vi "Refresh GMaps.vi"(0 "GMaps API in":refnum<class "GMaps API.lvclass">, 1 "Updating String":string, 2 "Automation Refnum in":refnum<k7>, 5 "error in (no error)":errorcluster, 6 "Google Maps API Key":string) -> (14 "GMaps API out":refnum<class "GMaps API.lvclass">, 15 "Updated String":string, 16 "Automation Refnum out":refnum<k7>, 19 "error out":errorcluster)   [LabVIEW 2016, in "GMaps API.lvclass"]
doc: "Refreshes the map when there is a new update of configuration options."
uses:
  GMaps API.lvclass
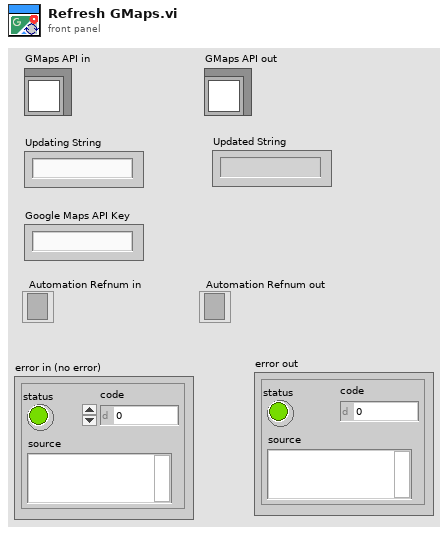
[diagram p1: front panel]
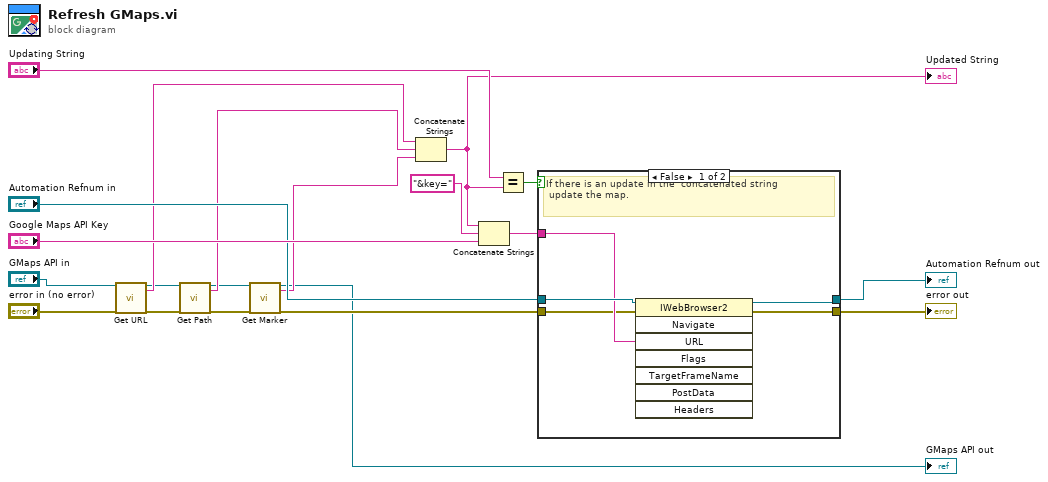
[diagram p0: block diagram]
diagram:
  n1 = call "Get URL.vi"("GMaps API in"="GMaps API in", "error in (no error)"="error in (no error)") -> ("GMaps API out"=w7:refnum<class "GMaps API.lvclass">, "Concateneted URL"=w12:string, "error out"=w5:errorcluster)  [unwired: 15 in]
  n2 = call "Get Path.vi"("GMaps API in"=w7, "error in (no error)"=w5) -> ("GMaps API out"=w6:refnum<class "GMaps API.lvclass">, "Concatenated Path"=w10:string, "error out"=w4:errorcluster)  [unwired: 15 in]
  n3 = call "Get Marker.vi"("GMaps API in"=w6, "error in (no error)"=w4) -> ("GMaps API out"=→"GMaps API out":refnum<class "GMaps API.lvclass">, "Concateneted Marker"=w11:string, "error out"=w3:errorcluster)  [unwired: 15 in]
  n4 = Concatenate Strings(w12, w10, w11) -> (w1:string)
  "Updated String" <- w1
  n5 = Concatenate Strings(w1, "&key=", "Google Maps API Key") -> (w20:string)
  n6 = Equal?(x="Updating String", y=w1) -> (x = y?=w15:bool)
  n7 = case shown="False" w15 {
    tunnel: "Automation Refnum in" -> [w25 w27]
    tunnel: [w24 w27] -> w14
    tunnel: w20 -> [w23 _]
    tunnel: w3 -> [w22 w26]
    tunnel: [w21 w26] -> w19
    frame False {
      # "If there is an update in the  concatenated string \n update the map."
      n8 = invoke class="IWebBrowser2" method="Navigate"(reference=w25, error in=w22, "URL"=w23) -> (reference out=w24:refnum<k7>, error out=w21:errorcluster)  [unwired: 5 in, 6 out]
    }
    frame True {
      # "If there is no update in the  concatenated string \ndo NOT update the map."
    }
  }
  "error out" <- w19
  "Automation Refnum out" <- w14
